vi "Write Data for averaging.vi"(8 "error in (no error)":errorcluster, 10 "Data for averaging":dbl[][](array[numeric]), 11 "Gage digitizer actor in":refnum<class "Gage digitizer actor.lvclass">) -> (0 "error out":errorcluster, 3 "Gage digitizer actor out":refnum<class "Gage digitizer actor.lvclass">)   [LabVIEW 2015, in "Gage digitizer actor.lvclass"]
uses:
  Gage digitizer actor.lvclass
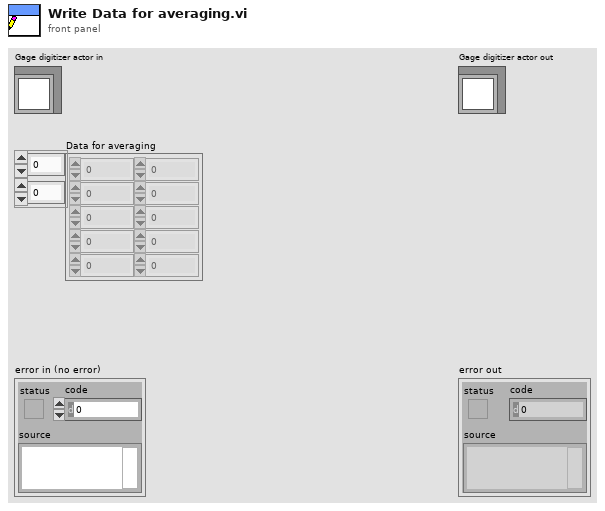
[diagram p1: front panel]
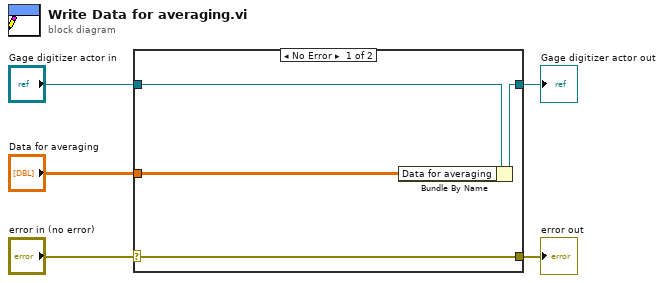
[diagram p0: block diagram]
diagram:
  n1 = case shown="No Error" "error in (no error)" {
    selector: "error in (no error)" -> [w9 w10]
    tunnel: [w9 w10] -> w4
    tunnel: [w7 w11] -> w2
    tunnel: "Gage digitizer actor in" -> [w8 w11]
    tunnel: "Data for averaging" -> [w6 _]
    frame No Error {
      n2 = Bundle By Name(cluster=w8, "Data for averaging"=w6) -> (w7:refnum<class "Gage digitizer actor.lvclass">)
    }
    frame Error {
    }
  }
  "error out" <- w4
  "Gage digitizer actor out" <- w2
